vi "filtr.vi"(8 "lower threshold":i32=1, 9 "upper threshold":i32=1, 11 "input array":dbl[][](array[numeric])) -> (3 "output array":dbl[][](array[numeric]))   [LabVIEW 2012]
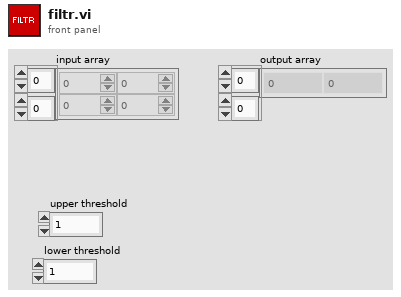
[diagram p1: front panel]
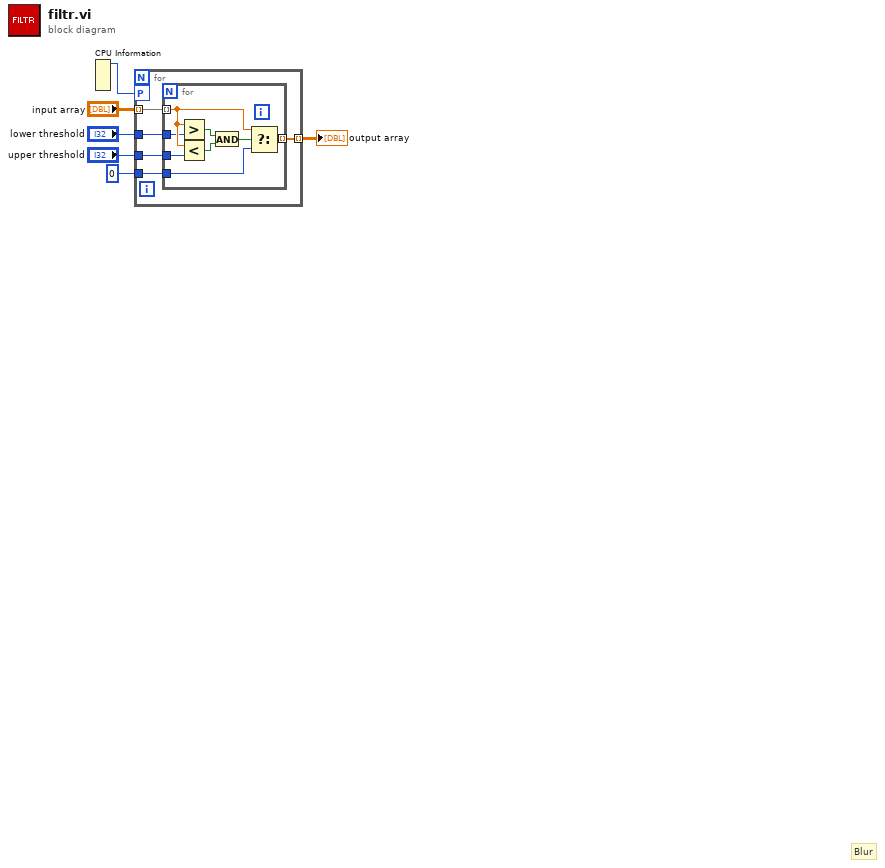
[diagram p0: block diagram]
diagram:
  # "Blur"
  n1 = CPU Information() -> (4:w2:i32)  [unwired: 3 out]
  n2 = for {
    tunnel: "input array" -> [w11] mode=indexing
    tunnel: "lower threshold" -> [w10]
    tunnel: [w9] -> w4 mode=indexing
    workers-P: w2 -> [_]
    tunnel: 0 -> [w8]
    tunnel: "upper threshold" -> [w7]
    n3 = for {
      tunnel: w11 -> [w17] mode=indexing
      tunnel: w10 -> [w15]
      tunnel: [w18] -> w9 mode=indexing
      tunnel: w8 -> [w19]
      tunnel: w7 -> [w16]
      n4 = Greater?(x=w17, y=w15) -> (0:w14:bool)
      n5 = Less?(x=w17, y=w16) -> (x < y?=w13:bool)
      n6 = And(x=w14, y=w13) -> (x .and. y?=w12:bool)
      n7 = Select(t=w17, s=w12, f=w19) -> (s? t:f=w18:dbl)
    }
  }
  "output array" <- w4
